vi "Tarea 4.vi"() -> ()   [LabVIEW 2019]
panel:
  out "Elapsed Time":dbl
  out "Bit 4":bool
  out "Bit 3":bool
  out "Bit 2":bool
  out "Bit 1":bool
  out "Time Has Elapsed":bool
  in  "Auto Reset":bool=TRUE
  in  "Reset Button":bool
  in  "Stop VI":bool
  in  "Time Target (s)":dbl=4.0
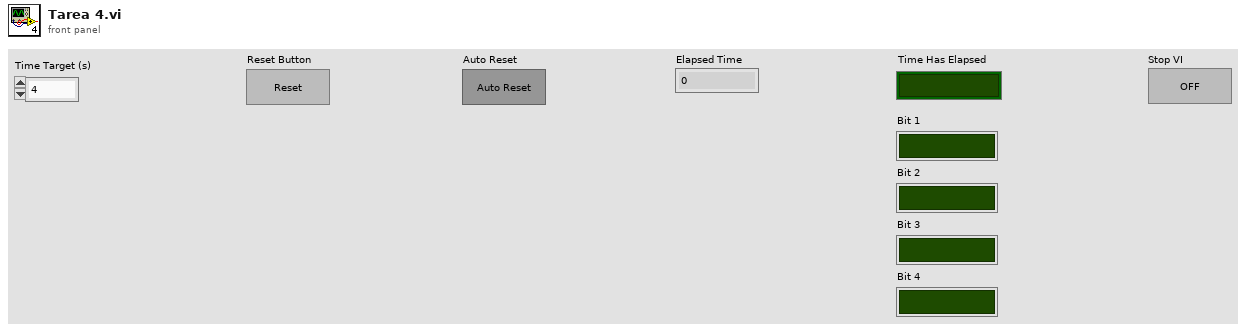
[diagram p1: front panel]
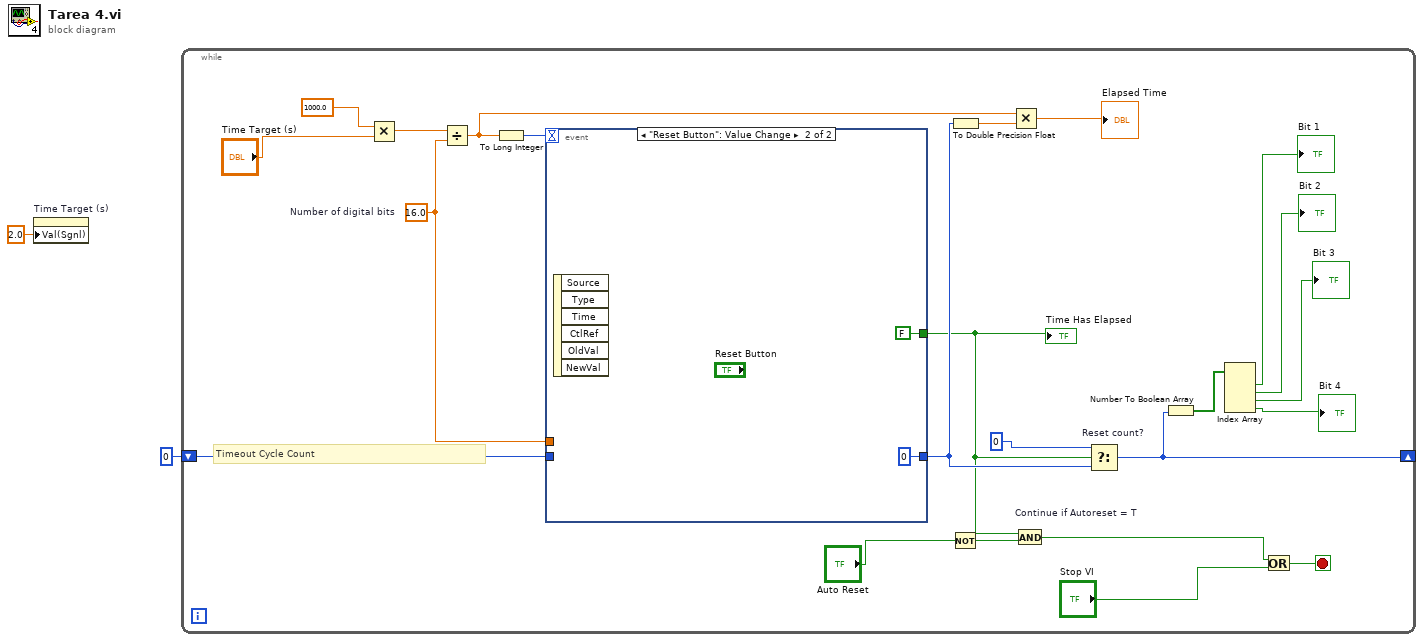
[diagram p0: block diagram]
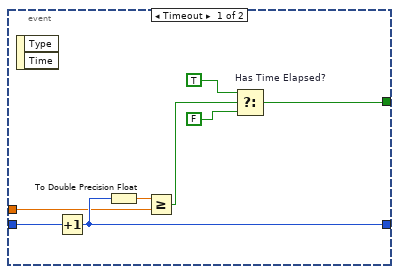
[diagram p2: hidden frame]
diagram:
  n1 = property on="Time Target (s)" class="DigNum (strict)"("Val(Sgnl)"=2.0 ("Value (Signaling)")) -> ()  [unwired: 2 in, 2 out]
  n2 = while {
    shift-right: [w15] -> _
    shift-left: 0 ("Reset Cycle Count") -> [w25]
    stop <- w21 stop-if-true
    w14 = 16.0  # Number of digital bits
    # "Timeout Cycle Count"
    n3 = Multiply(x=1000.0, y="Time Target (s)") -> (x*y=w23:dbl)
    n4 = Divide(x=w23, y=w14) -> (x/y=w19:dbl)
    n5 = To Long Integer(number=w19) -> (32bit integer=w12:i32)
    n6 = event shown="[1] \"Reset Button\": Value Change" {
      selector: _ -> [_ _]
      dyn-events: _ -> [_ _]
      timeout: w12 -> [_ _]
      tunnel: [w28 0 ("Reset Cycle Count")] -> w16
      tunnel: w25 -> [w33 _]
      tunnel: [w29 FALSE] -> w3
      tunnel: w14 -> [w27 _]
      event Timeout {
        n7 = event-data() -> ()  [unwired: 1 in, 2 out]
        n8 = Increment(x=w33) -> (x+1=w28:i32)
        n9 = To Double Precision Float(number=w28) -> (double precision float=w26:dbl)
        n10 = Greater Or Equal?(x=w26, y=w27) -> (x >= y?=w32:bool)
        n11 = Select "Has Time Elapsed?"(t=TRUE, s=w32, f=FALSE) -> (s? t:f=w29:bool)
      }
      event "Reset Button": Value Change {
        n12 = event-data() -> ()  [unwired: 1 in, 6 out]
      }
    }
    "Time Has Elapsed" <- w3
    n13 = Not(x="Auto Reset") -> (.not. x?=w18:bool)
    n14 = To Double Precision Float(number=w16) -> (double precision float=w13:dbl)
    n15 = Multiply(x=w19, y=w13) -> (x*y=→"Elapsed Time":dbl)
    n16 = And "Continue if Autoreset = T"(x=w3, y=w18) -> (x .and. y?=w20:bool)
    n17 = Select "Reset count?"(t=0, s=w3, f=w16) -> (s? t:f=w15:i32)
    n18 = Number To Boolean Array(number=w15) -> (Boolean array=w24:bool[])
    n19 = Index Array(array=w24) -> (element #1=→"Bit 1":bool, element #2=→"Bit 2":bool, element #3=→"Bit 3":bool, element #4=→"Bit 4":bool)  [unwired: 4 in]
    n20 = Or(x=w20, y="Stop VI") -> (x .or. y?=w21:bool)
  }
